vi "Create OPC UA Client.vi"(8 "error in (no error)":errorcluster, 9 "update rate (1000 ms)":dbl=1000.0, 10 "port (4840)":i32=4840, 11 "URLs":string[](array[string])) -> (0 "error out":errorcluster, 1 "subscription ID out":u32, 2 "OPC UA client refnum out":refnum<k21>, 3 "OPC UA data change event":refnum<user-event>)   [LabVIEW 2015]
uses:
  <vilib>/OPCUA/NI OPC UA Client.lvlib
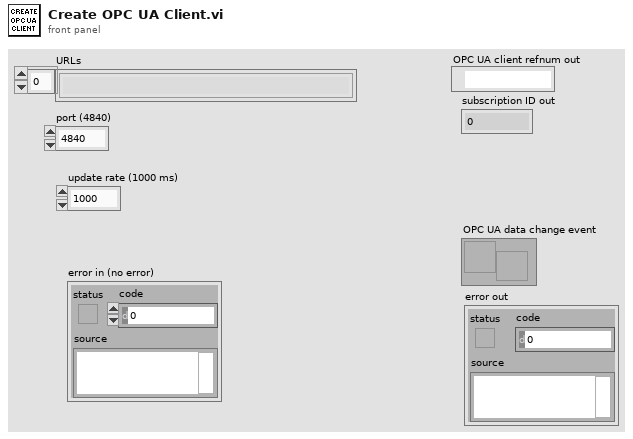
[diagram p1: front panel]
types:
  T1 = cluster{"message mode":enum16{"None", "Sign", "Sign and Encrypt"}, "security":enum16{"Basic256", "Basic128Rsa15"}}
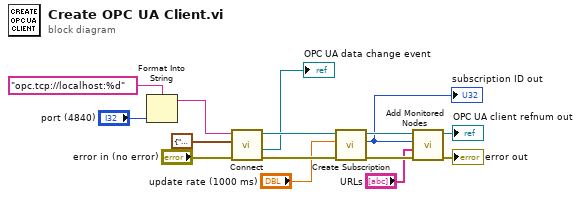
[diagram p0: block diagram]
diagram:
  n1 = Format Into String(format string="opc.tcp://localhost:%d" ("server endpoint URL"), "port (4840)") -> (resulting string=w12:string)  [unwired: 2 in, 1 out]
  n2 = call <vilib>:"Connect.vi"("error in (no error)"="error in (no error)", "security policy"=T1 {"message mode"=enum."None", "security"=enum."Basic256"}, "server endpoint URL"=w12) -> ("error out"=w11:errorcluster, "OPC UA data change event"=→"OPC UA data change event":refnum<user-event>, "OPC UA client refnum out"=w9:refnum<k21>)  [unwired: 6 in]
  n3 = call <vilib>:"Create Subscription.vi"("error in (no error)"=w11, "update rate (1000 ms)"="update rate (1000 ms)", "OPC UA client refnum in"=w9) -> ("error out"=w14:errorcluster, "subscription ID out"=w7:u32, "OPC UA client refnum out"=w15:refnum<k21>)  [unwired: 6 in]
  "subscription ID out" <- w7
  n4 = call <vilib>:"Add Monitored Nodes.vi"("error in (no error)"=w14, "array of node path"="URLs", "subscription ID in"=w7, "OPC UA client refnum in"=w15) -> ("error out"=→"error out":errorcluster, "OPC UA client refnum out"=→"OPC UA client refnum out":refnum<k21>)  [unwired: 5 in, 1 out]
